vi "DSF.Engine.Framework.Initialize.Transfer Groups.Sort Rx and Tx by Priority.vi"(8 "error in (no error)":errorcluster, 11 "Framework in":refnum<class "Framework.lvclass">) -> (0 "error out":errorcluster, 3 "Framework out":refnum<class "Framework.lvclass">)   [LabVIEW 2017, in "DSF.Engine.lvlib" / "Framework.lvclass"]
uses:
  Framework.lvclass
  Framework.lvclass/Framework.ctl
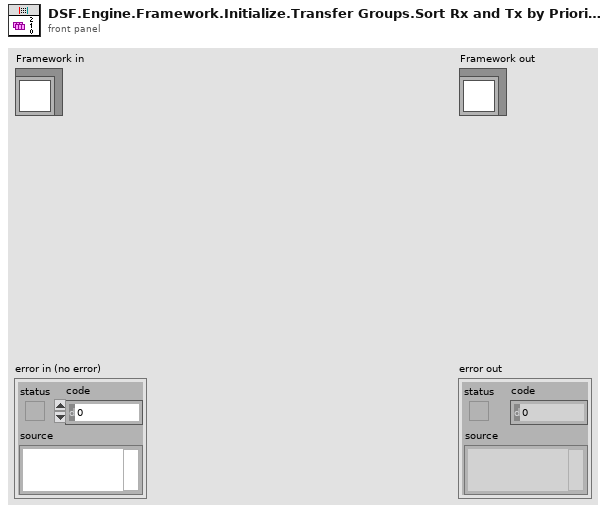
[diagram p1: front panel]
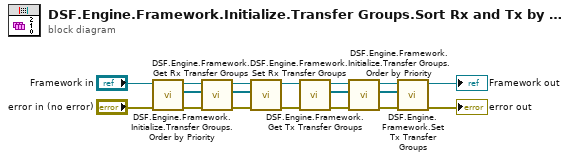
[diagram p0: block diagram]
diagram:
  n1 = call "DSF.Engine.Framework.Get Rx Transfer Groups.vi"("Framework in"="Framework in") -> ("Rx Transfer Groups"=w12:refnum<class "DSF.Engine.Transfer Group.lvclass">[], "Framework out"=w13:refnum<class "Framework.lvclass">)  [unwired: 9 in]
  n2 = call "DSF.Engine.Framework.Initialize.Transfer Groups.Order by Priority.vi"("error in (no error)"="error in (no error)", "Transfer Groups"=w12, "Framework in"=w13) -> ("error out"=w5:errorcluster, "sorted Transfer Groups"=w10:refnum<class "DSF.Engine.Transfer Group.lvclass">[], "Framework out"=w11:refnum<class "Framework.lvclass">)  [unwired: 6 in]
  n3 = call "DSF.Engine.Framework.Set Rx Transfer Groups.vi"("Rx Transfer Groups"=w10, "Framework in"=w11) -> ("Framework out"=w8:refnum<class "Framework.lvclass">)  [unwired: 9 in]
  n4 = call "DSF.Engine.Framework.Get Tx Transfer Groups.vi"("Framework in"=w8) -> ("Tx Transfer Groups"=w6:refnum<class "DSF.Engine.Transfer Group.lvclass">[], "Framework out"=w7:refnum<class "Framework.lvclass">)  [unwired: 9 in]
  n5 = call "DSF.Engine.Framework.Initialize.Transfer Groups.Order by Priority.vi"("error in (no error)"=w5, "Transfer Groups"=w6, "Framework in"=w7) -> ("error out"=→"error out":errorcluster, "sorted Transfer Groups"=w4:refnum<class "DSF.Engine.Transfer Group.lvclass">[], "Framework out"=w3:refnum<class "Framework.lvclass">)  [unwired: 6 in]
  n6 = call "DSF.Engine.Framework.Set Tx Transfer Groups.vi"("Tx Transfer Groups"=w4, "Framework in"=w3) -> ("Framework out"=→"Framework out":refnum<class "Framework.lvclass">)  [unwired: 9 in]
